vi "OCR_Determine column type from colors.vi"(4 "Seperator Or Letter If Solid":bool, 6 "Color Set":T1={"BG"=255, "FG"=16711680}, 8 "Error":errorcluster, 11 "Color List":u32[](array[colorbox])) -> (0 "Error Out":errorcluster, 3 "Type Out":T2)   [LabVIEW 2009]
doc: "Determines the Column type from the color list"
uses:
  Controls/Enum/ENUM_Line Letter Type.ctl
  Controls/Cluster/Cluster_Text Color Set.ctl
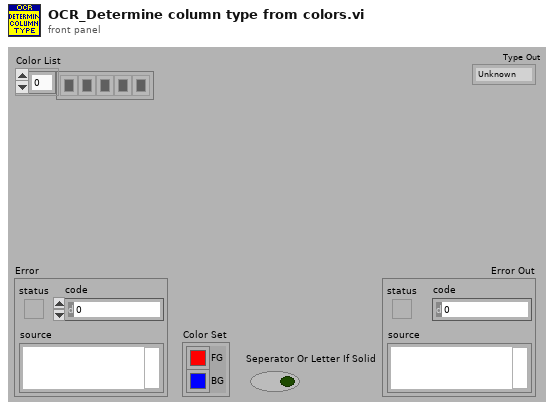
[diagram p1: front panel]
types:
  T1 = typedef "Cluster_Text Color Set.ctl" = cluster{"BG":u32, "FG":u32}
  T2 = typedef "ENUM_Line Letter Type.ctl" = enum16{"Unknown", "Letter", "Seperator", "Seperator or Letter"}
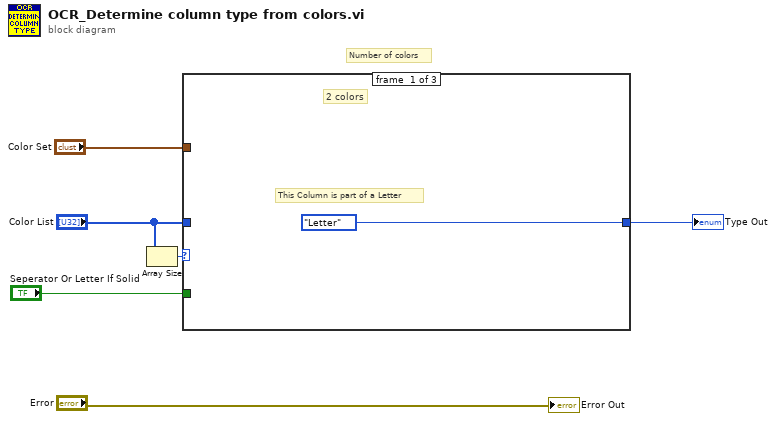
[diagram p0: block diagram]
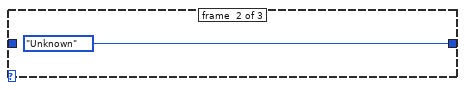
[diagram p2: hidden frame]
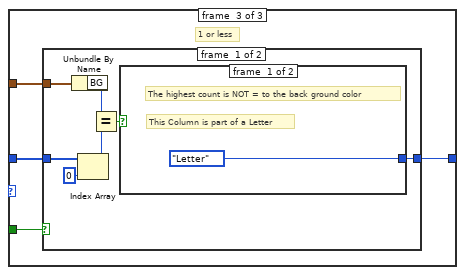
[diagram p3: hidden frame]
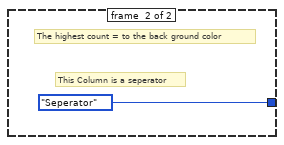
[diagram p4: hidden frame]
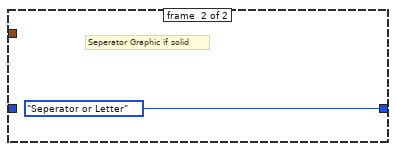
[diagram p5: hidden frame]
diagram:
  # "Number of colors"
  n1 = Array Size(array="Color List") -> (size(s)=w3:i32)
  n2 = case shown="..1" w3 {
    tunnel: [ENUM_Line_Letter_Type."Letter" ("Type Out") ENUM_Line_Letter_Type."Unknown" ("Type Out") w12] -> w5
    tunnel: "Color List" -> [_ _ w10]
    tunnel: "Color Set" -> [_ _ w11]
    tunnel: "Seperator Or Letter If Solid" -> [_ _ w9]
    frame #0 {
      # "This Column is part of a Letter"
      # "2 colors"
    }
    frame #1 {
    }
    frame #2 {
      # "1 or less"
      n3 = case shown="True" w9 {
        tunnel: [w19 ENUM_Line_Letter_Type."Seperator or Letter" ("Type Out")] -> w12
        tunnel: w11 -> [w18 _]
        tunnel: w10 -> [w17 _]
        frame #0 {
          n4 = Unbundle By Name(w18) -> ("BG"=w15:u32)
          n5 = Index Array(array=w17, index=0) -> (element=w14:u32)
          n6 = Equal?(x=w15, y=w14) -> (x = y?=w13:bool)
          n7 = case shown="True" w13 {
            tunnel: [ENUM_Line_Letter_Type."Letter" ("Type Out") ENUM_Line_Letter_Type."Seperator" ("Type Out")] -> w19
            frame #0 {
              # "This Column is part of a Letter"
              # "The highest count is NOT = to the back ground color"
            }
            frame #1 {
              # "This Column is a seperator"
              # "The highest count = to the back ground color"
            }
          }
        }
        frame #1 {
          # "Seperator Graphic if solid"
        }
      }
    }
  }
  "Type Out" <- w5
  "Error Out" <- "Error"
